vi "term_op.vi"() -> ()   [LabVIEW 2020]
panel:
  out "Waveform Chart":dynamicdata(graph)
  out "Numeric 7":dbl
  out "Numeric 6":dbl
  out "Numeric 5":dbl
  out "Numeric 4":dbl
  out "Numeric 3":dbl
  out "Numeric 2":dbl
  out "Numeric":dbl
  in  "stop":bool
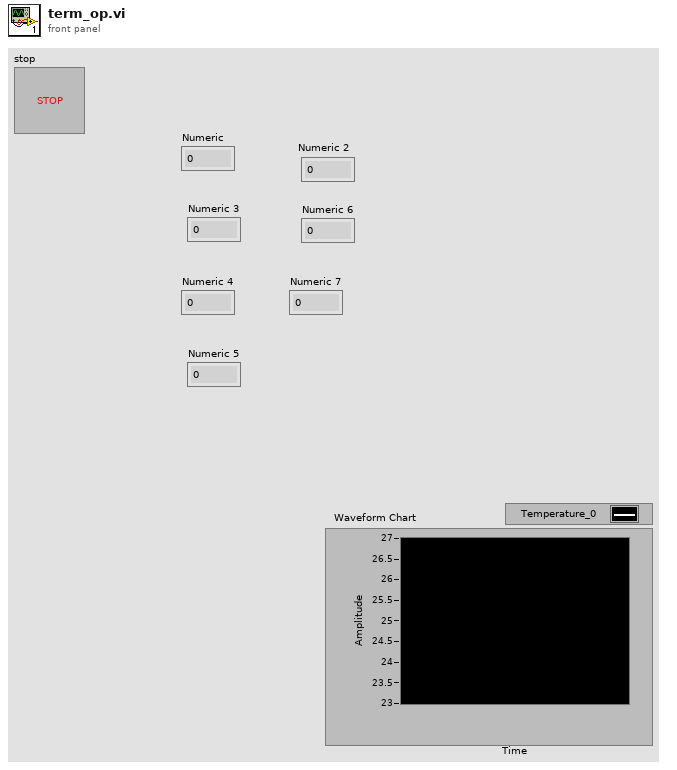
[diagram p1: front panel]
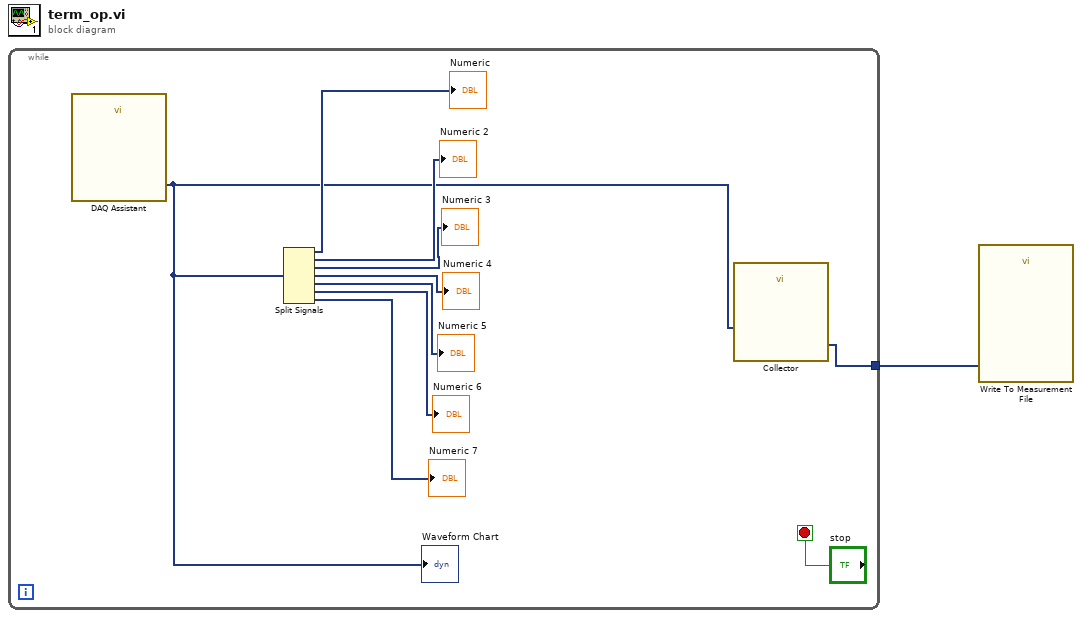
[diagram p0: block diagram]
diagram:
  n1 = while {
    tunnel: [w2] -> w1
    stop <- "stop" stop-if-true
    n2 = call "DAQ Assistant"() -> ("data"=w3:dynamicdata)  [unwired: 16 in, 3 out]
    "Waveform Chart" <- w3
    n3 = Split Signals(w3) -> (→"Numeric":dynamicdata, →"Numeric 2":dynamicdata, →"Numeric 3":dynamicdata, →"Numeric 4":dynamicdata, →"Numeric 5":dynamicdata, →"Numeric 6":dynamicdata, →"Numeric 7":dynamicdata)  [unwired: 7 in]
    n4 = call "Collector"("Signals"=w3) -> ("Collected Signals"=w2:dynamicdata)  [unwired: 9 in, 1 out]
  }
  n5 = call "Write To Measurement File"("Signals"=w1) -> ()  [unwired: 16 in, 3 out]
